vi "test Adjust Text to Fit Rectangle.vi"(11 "Test Case In":refnum<class "test Adjust Text to Fit Rectangle.lvclass">) -> (0 "error out":errorcluster, 3 "Test Case Out":refnum<class "test Adjust Text to Fit Rectangle.lvclass">)   [LabVIEW 2020, in "test Adjust Text to Fit Rectangle.lvclass"]
uses:
  test Adjust Text to Fit Rectangle.lvclass
  C:/Program Files/National Instruments/LabVIEW 2026/vi.lib/Astemes/LUnit/Test Case.lvclass
  <vilib>/Astemes/LUnit/Test Case.lvclass/Test Case.ctl
  <vilib>/LabVIEW Icon API/API_Text.ctl
  <vilib>/LabVIEW Icon API/LabVIEW Icon API.lvlib
  <vilib>/LabVIEW Icon API/Set Text Icon/Text-Based VI Icon.lvlib
  <vilib>/LabVIEW Icon API/API_Text Colors.ctl
  <vilib>/LabVIEW Icon API/lv_icon/Controls/Alignment.ctl
  <vilib>/LabVIEW Icon API/API_Test Settings.ctl
  <vilib>/Astemes/LUnit/Test Case.lvclass
panel:
  out "NOKs":T1[](array[typedef])
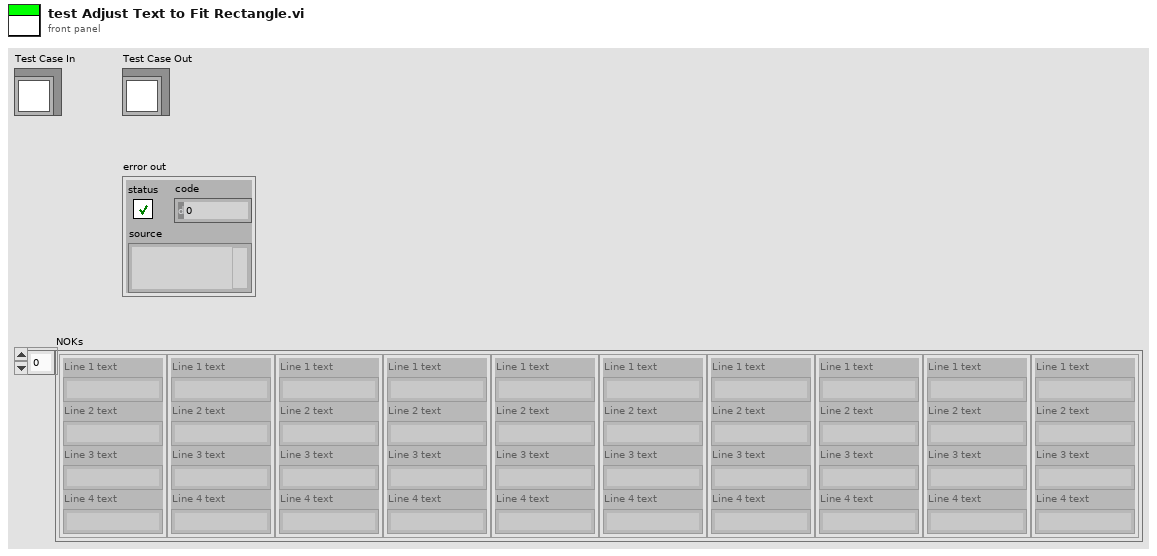
[diagram p1: front panel]
types:
  T1 = typedef "LabVIEW Icon API.lvlib/API_Text.ctl" = cluster{"Line 1 text":string, "Line 2 text":string, "Line 3 text":string, "Line 4 text":string}
  T2 = typedef "LabVIEW Icon API.lvlib/API_Test Settings.ctl" = cluster{"Font":string, "Alignment":T3, "Size":u8, "Center text":bool, "Capitalize text":bool, "Text color":T4}
  T3 = typedef "Alignment.ctl" = u16
  T4 = typedef "LabVIEW Icon API.lvlib/API_Text Colors.ctl" = cluster{"Line 1 color":u32, "Line 2 color":u32, "Line 3 color":u32, "Line 4 color":u32}
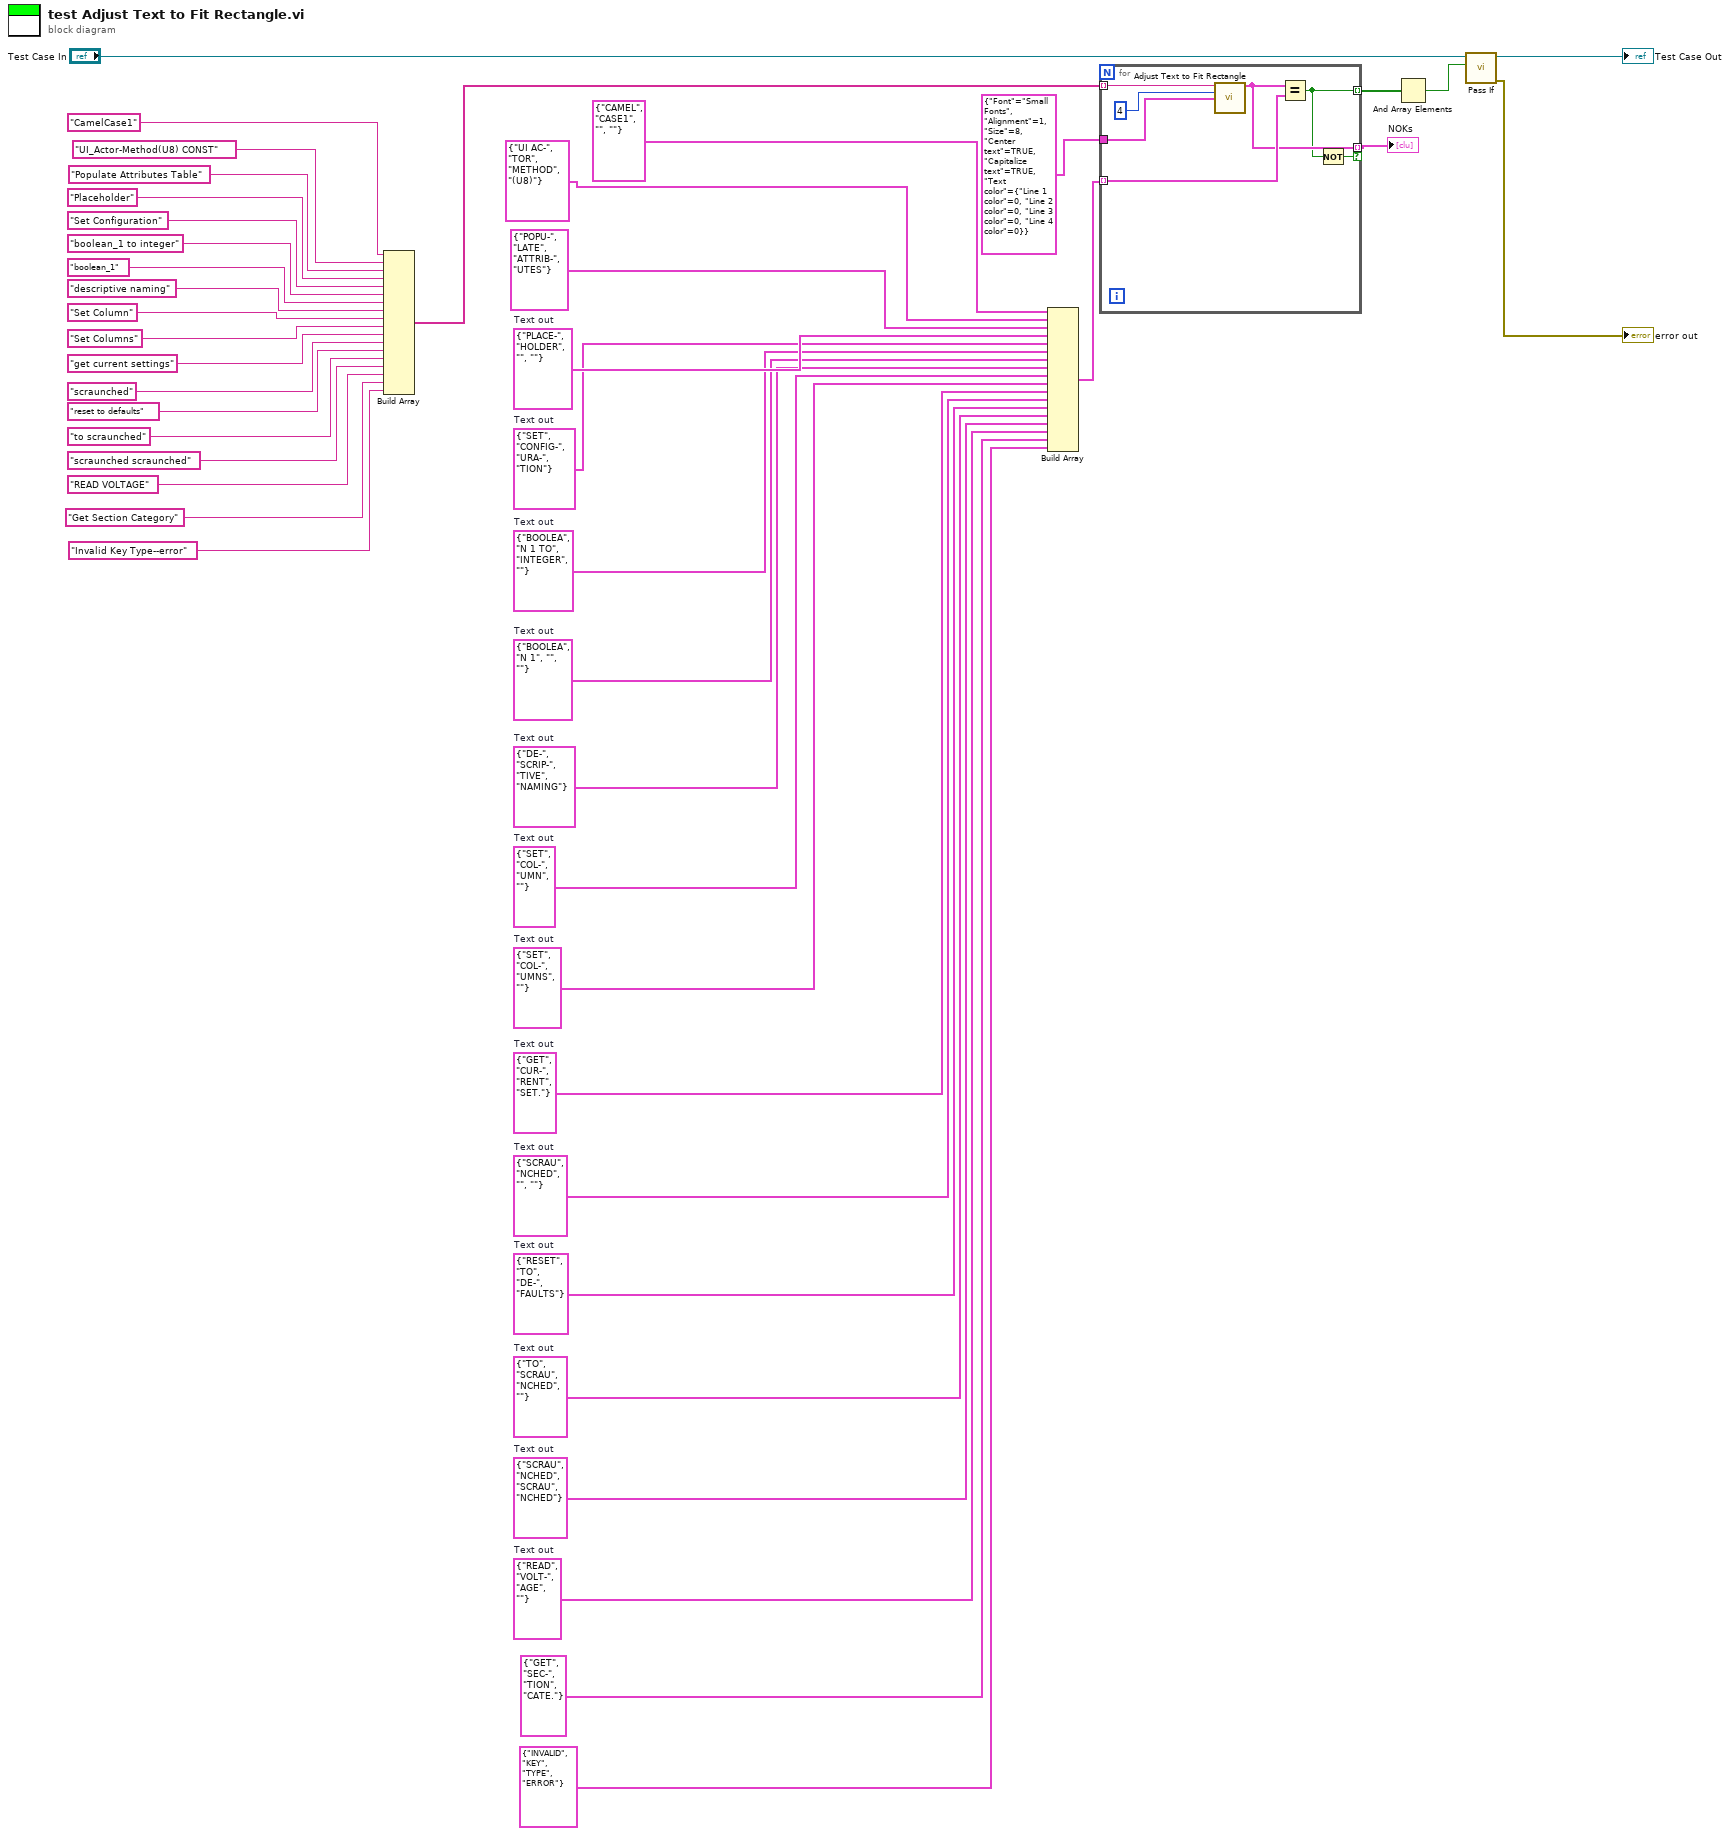
[diagram p0: block diagram]
diagram:
  w17 = T1 {"Line 1 text"="READ", "Line 2 text"="VOLT-", "Line 3 text"="AGE", "Line 4 text"=""}  # Text out
  w18 = T1 {"Line 1 text"="SCRAU", "Line 2 text"="NCHED", "Line 3 text"="SCRAU", "Line 4 text"="NCHED"}  # Text out
  w19 = T1 {"Line 1 text"="TO", "Line 2 text"="SCRAU", "Line 3 text"="NCHED", "Line 4 text"=""}  # Text out
  w20 = T1 {"Line 1 text"="RESET", "Line 2 text"="TO", "Line 3 text"="DE-", "Line 4 text"="FAULTS"}  # Text out
  w21 = T1 {"Line 1 text"="SCRAU", "Line 2 text"="NCHED", "Line 3 text"="", "Line 4 text"=""}  # Text out
  w22 = T1 {"Line 1 text"="GET", "Line 2 text"="CUR-", "Line 3 text"="RENT", "Line 4 text"="SET."}  # Text out
  w23 = T1 {"Line 1 text"="SET", "Line 2 text"="COL-", "Line 3 text"="UMNS", "Line 4 text"=""}  # Text out
  w24 = T1 {"Line 1 text"="SET", "Line 2 text"="COL-", "Line 3 text"="UMN", "Line 4 text"=""}  # Text out
  w25 = T1 {"Line 1 text"="DE-", "Line 2 text"="SCRIP-", "Line 3 text"="TIVE", "Line 4 text"="NAMING"}  # Text out
  w26 = T1 {"Line 1 text"="BOOLEA", "Line 2 text"="N 1", "Line 3 text"="", "Line 4 text"=""}  # Text out
  w27 = T1 {"Line 1 text"="BOOLEA", "Line 2 text"="N 1 TO", "Line 3 text"="INTEGER", "Line 4 text"=""}  # Text out
  w28 = T1 {"Line 1 text"="SET", "Line 2 text"="CONFIG-", "Line 3 text"="URA-", "Line 4 text"="TION"}  # Text out
  w29 = T1 {"Line 1 text"="PLACE-", "Line 2 text"="HOLDER", "Line 3 text"="", "Line 4 text"=""}  # Text out
  n1 = Build Array("CamelCase1" ("element"), "UI_Actor-Method(U8) CONST" ("element"), "Populate Attributes Table" ("element"), "Placeholder" ("Input"), "Set Configuration" ("Input"), "boolean_1 to integer" ("Input"), "boolean_1" ("Input"), "descriptive naming" ("Input"), "Set Column" ("Input"), "Set Columns" ("Input"), "get current settings" ("Input"), "scraunched" ("Input"), "reset to defaults" ("Input"), "to scraunched" ("Input"), "scraunched scraunched" ("Input"), "READ VOLTAGE" ("Input"), "Get Section Category" ("element"), "Invalid Key Type--error" ("element")) -> (w16:string[])
  n2 = Build Array(T1 {"Line 1 text"="CAMEL", "Line 2 text"="CASE1", "Line 3 text"="", "Line 4 text"=""} ("element"), T1 {"Line 1 text"="UI AC-", "Line 2 text"="TOR", "Line 3 text"="METHOD", "Line 4 text"="(U8)"} ("Text out"), T1 {"Line 1 text"="POPU-", "Line 2 text"="LATE", "Line 3 text"="ATTRIB-", "Line 4 text"="UTES"} ("element"), w29, w28, w27, w26, w25, w24, w23, w22, w21, w20, w19, w18, w17, T1 {"Line 1 text"="GET", "Line 2 text"="SEC-", "Line 3 text"="TION", "Line 4 text"="CATE."} ("element"), T1 {"Line 1 text"="INVALID", "Line 2 text"="KEY", "Line 3 text"="TYPE", "Line 4 text"="ERROR"} ("element")) -> (w14:T1[])
  n3 = for {
    tunnel: w16 -> [w52] mode=indexing
    tunnel: T2 {"Font"="Small Fonts", "Alignment"=1, "Size"=8, "Center text"=TRUE, "Capitalize text"=TRUE, "Text color"={"Line 1 color"=0, "Line 2 color"=0, "Line 3 color"=0, "Line 4 color"=0}} ("Text settings") -> [w51]
    tunnel: w14 -> [w50] mode=indexing
    tunnel: [w46] -> w13 mode=indexing
    tunnel: [w48] -> w5 mode=indexing if=w47
    n4 = call "Adjust Text to Fit Rectangle.vi"("VI Name"=w52, "Number of Rows"=4, "Text settings"=w51) -> ("Text out"=w48:T1)  [unwired: 12 in]
    n5 = Equal?(x=w48, y=w50) -> (x = y?=w46:bool)
    n6 = Not(x=w46) -> (.not. x?=w47:bool)
  }
  "NOKs" <- w5
  n7 = And Array Elements(Boolean array=w13) -> (logical AND=w12:bool)
  n8 = call <vilib>:"Pass If.vi"("Pass?"=w12, "LUnit Test Case In"="Test Case In") -> ("error out"=→"error out":errorcluster, "LUnit Test Case Out"=→"Test Case Out":refnum<class "test Adjust Text to Fit Rectangle.lvclass">)  [unwired: 8 in]
